vi "Determine warnings. vi.vi"() -> ()   [LabVIEW 2014]
panel:
  out "Warning":bool
  out "Warning Text":string
  in  "Min Temp":dbl
  in  "Max Temp":dbl
  in  "Current Temp":dbl
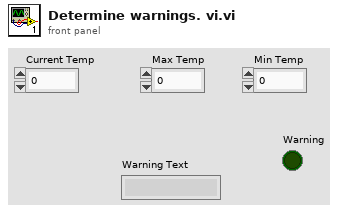
[diagram p1: front panel]
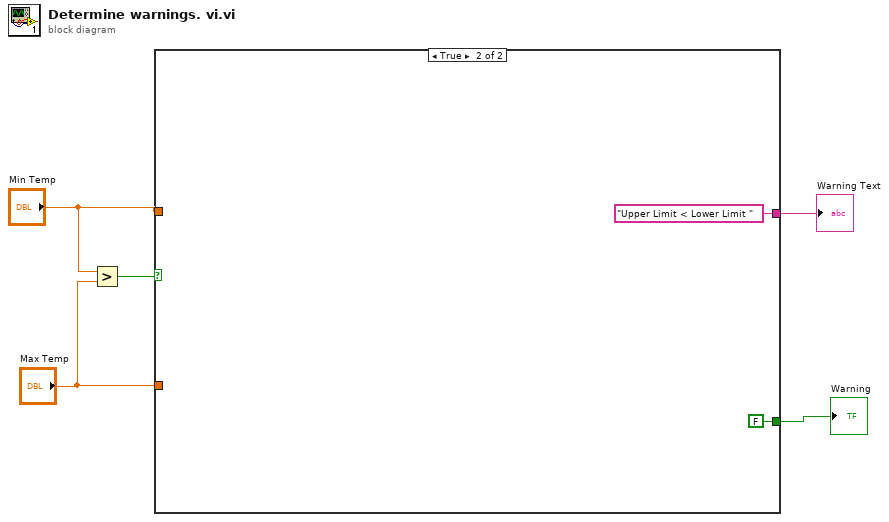
[diagram p0: block diagram]
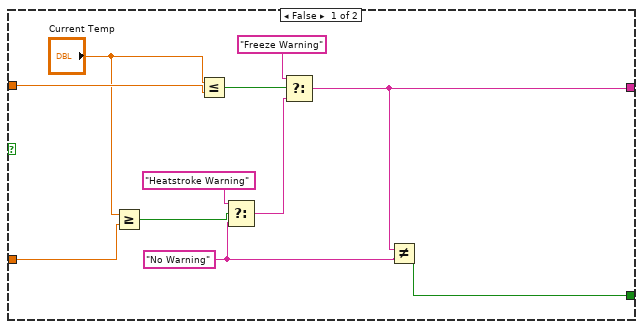
[diagram p2: hidden frame]
diagram:
  n1 = Greater?(x="Min Temp", y="Max Temp") -> (0:w3:bool)
  n2 = case shown="True" w3 {
    tunnel: "Max Temp" -> [w7 _]
    tunnel: "Min Temp" -> [w9 _]
    tunnel: [w16 FALSE] -> w5
    tunnel: [w11 "Upper Limit < Lower Limit "] -> w4
    frame False {
      w12 = "No Warning"
      n3 = Greater Or Equal?(x="Current Temp", y=w7) -> (x >= y?=w8:bool)
      n4 = Less Or Equal?(x="Current Temp", y=w9) -> (x <= y?=w10:bool)
      n5 = Select(t="Heatstroke Warning", s=w8, f=w12) -> (s? t:f=w14:string)
      n6 = Select(t="Freeze Warning", s=w10, f=w14) -> (s? t:f=w11:string)
      n7 = Not Equal?(x=w11, y=w12) -> (x != y?=w16:bool)
    }
    frame True {
    }
  }
  "Warning Text" <- w4
  "Warning" <- w5
